vi "Server 2 - Copy2.vi"() -> ()   [LabVIEW 2017]
uses:
  <vilib>/Analysis/Matrix/Datatypes/RealMatrix.ctl
  <vilib>/Analysis/Matrix/Numeric/Multiply/Multiply - RM,RM.vi
  <vilib>/Analysis/Matrix/NI_Matrix.lvlib
panel:
  out "RESULT":T1
  in  "MATRIX FROM SERVER":T1
  out "MATRIX FROM CLIENT":T1
  in  "Real Matrix":T1
  out "DATA FROM CLIENT":i32
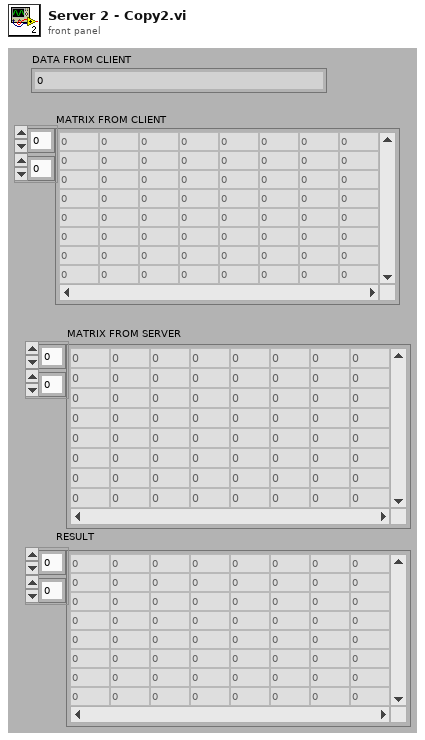
[diagram p1: front panel]
types:
  T1 = typedef "NI_Matrix.lvlib/RealMatrix.ctl" = dbl[][]
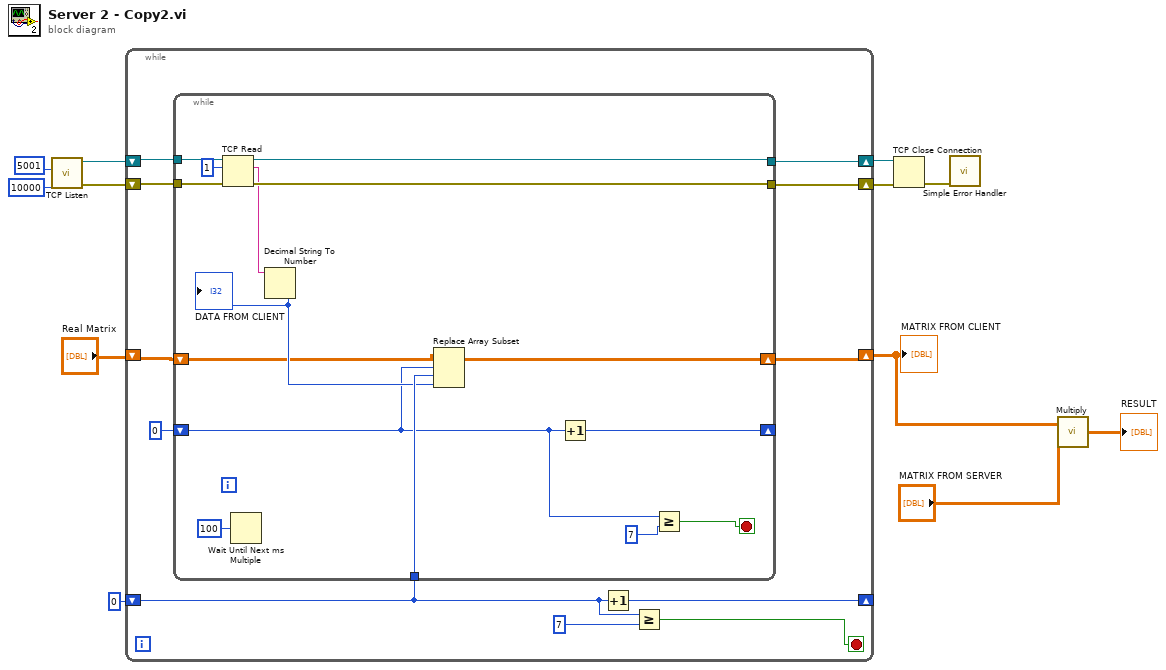
[diagram p0: block diagram]
diagram:
  n1 = call <vilib>:"TCP Listen.vi"("timeout ms (wait forever: -1)"=10000, "port"=u16 5001) -> ("error out"=w11:errorcluster, "connection ID"=w12:refnum<k5>)  [unwired: 5 in, 3 out]
  n2 = while {
    shift-right: [w21] -> w5
    shift-left: w12 -> [w23]
    shift-right: [w20] -> w10
    shift-left: w11 -> [w22]
    shift-right: [w19] -> _
    shift-left: u32 0 ("millisecond multiple") -> [w17]
    shift-right: [w13] -> w2
    shift-left: "Real Matrix" -> [w14]
    stop <- w15 stop-if-true
    n3 = while {
      tunnel: w23 -> [w38]
      tunnel: w22 -> [w37]
      tunnel: [w35] -> w21
      tunnel: [w33] -> w20
      tunnel: w17 -> [w31]
      shift-right: [w30] -> _
      shift-left: u32 0 ("millisecond multiple") -> [w27]
      shift-right: [w24] -> w13
      shift-left: w14 -> [w25]
      stop <- w28 stop-if-true
      n4 = TCP Read(connection ID=w38, bytes to read=1, error in (no error)=w37) -> (connection ID out=w35:refnum<k5>, data out=w32:string, error out=w33:errorcluster)  [unwired: 2 in]
      n5 = Wait Until Next ms Multiple(millisecond multiple=u32 100) -> ()  [unwired: 1 out]
      n6 = Decimal String To Number(string=w32) -> (number=w29:i32)  [unwired: 2 in, 1 out]
      "DATA FROM CLIENT" <- w29
      n7 = Replace Array Subset(array=w25, new element=w29, index (row)=w27, index (col)=w31) -> (w24:T1)
      n8 = Increment(x=w27) -> (x+1=w30:u32)
      n9 = Greater Or Equal?(x=w27, y=u32 7 ("millisecond multiple")) -> (x >= y?=w28:bool)
    }
    n10 = Increment(x=w17) -> (x+1=w19:u32)
    n11 = Greater Or Equal?(x=w17, y=u32 7 ("millisecond multiple")) -> (x >= y?=w15:bool)
  }
  "MATRIX FROM CLIENT" <- w2
  n12 = TCP Close Connection(connection ID=w5, error in (no error)=w10) -> (error out=w4:errorcluster)  [unwired: 1 in, 1 out]
  n13 = call <vilib>:"Simple Error Handler.vi"("error in (no error)"=w4) -> ()  [unwired: 4 in, 5 out]
  n14 = call-poly <vilib>:"Multiply.vi"("Real Matrix B"="MATRIX FROM SERVER", "Real Matrix A"=w2) -> ("A * B"=→"RESULT":T1)
